vi "FileIO-Circular Wav Read.vi"(0 "Fileref in":T1, 5 "stimfileend":bool, 7 "Nread":i32, 9 "Loop?":bool, 11 "error in (no error)":errorcluster) -> (4 "Fileref out":T1, 6 "end of file?":bool, 8 "Y":dbl[](array[numeric]), 10 "looped":bool, 15 "error out":errorcluster)   [LabVIEW 2020]
uses:
  <vilib>/sound2/lvsound2.llb/Sound File Refnum.ctl
  <vilib>/sound2/lvsound2.llb/Sound File Position.ctl
  <vilib>/sound2/lvsound2.llb/Sound File Read (DBL).vi
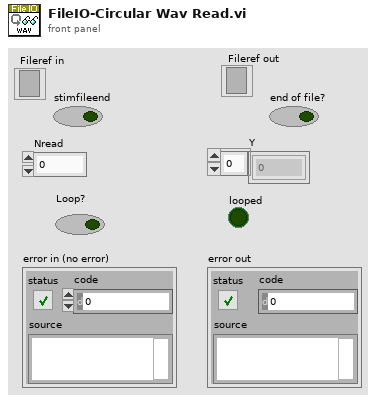
[diagram p1: front panel]
types:
  T1 = typedef "Sound File Refnum.ctl" = refnum<file>
  T2 = typedef "Sound File Position.ctl" = u16
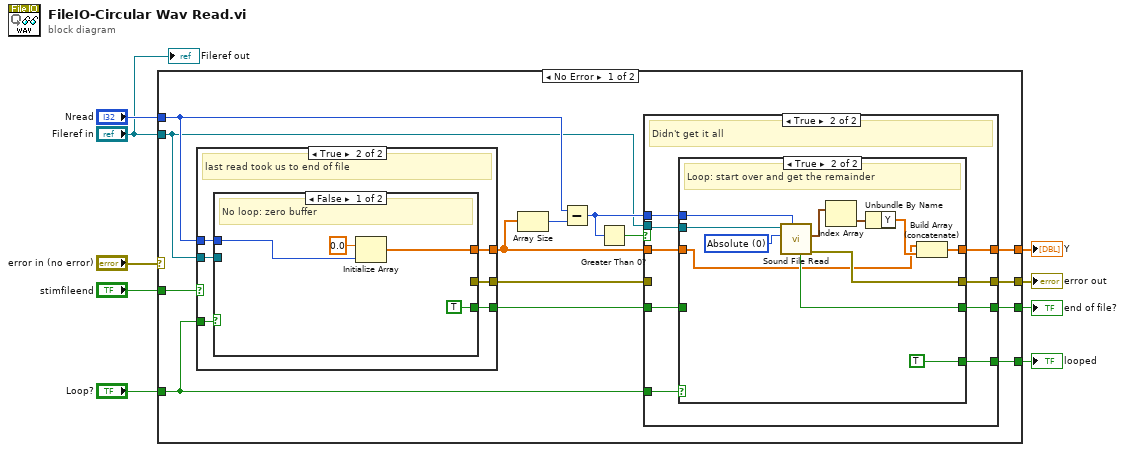
[diagram p0: block diagram]
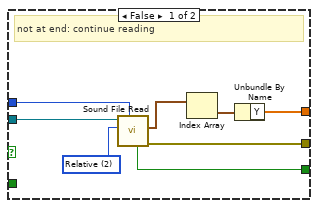
[diagram p2: hidden frame]
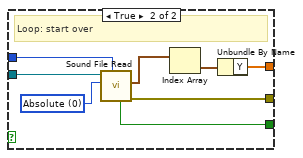
[diagram p3: hidden frame]
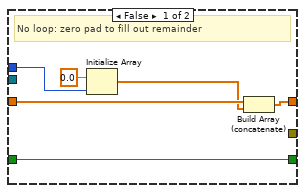
[diagram p5: hidden frame]
diagram:
  n1 = case shown="No Error" "error in (no error)" {
    selector: "error in (no error)" -> [_ w79]
    tunnel: "stimfileend" -> [w23 _]
    tunnel: "Nread" -> [w21 _]
    tunnel: "Fileref in" -> [w14 _]
    tunnel: "Loop?" -> [w13 _]
    tunnel: [w18 _] -> w4
    tunnel: [w16 w79] -> w3
    tunnel: [w11 _] -> w2
    tunnel: [w10 _] -> w1
    frame No Error {
      n2 = case shown="True" w23 {
        tunnel: [w26 w37] -> w17
        tunnel: w21 -> [w27 w36]
        tunnel: w14 -> [w28 w35]
        tunnel: w13 -> [_ w34]
        tunnel: [w25 w33] -> w19
        tunnel: [w24 w32] -> w12
        frame False {
          w31 = T2 2 items=["Absolute"=0, "Relative"=2] ("position mode")
          # "not at end: continue reading"
          n3 = call-poly <vilib>:"Sound File Read.vi"("number of samples/ch (-1: all)"=w27, "position mode"=w31, "sound file refnum"=w28) -> ("error out"=w26:errorcluster, "data"=w29:waveform(dbl)[], "end of file?"=w24:bool)  [unwired: 4 in, 2 out]
          n4 = Index Array(array=w29) -> (element=w30:waveform(dbl))  [unwired: 1 in]
          n5 = Unbundle By Name(w30) -> ("Y"=w25:dbl[])
        }
        frame True {
          # "last read took us to end of file"
          n6 = case shown="False" w34 {
            tunnel: [TRUE ("end of file?") w49] -> w32
            tunnel: [_ w48] -> w37
            tunnel: w36 -> [w41 w47]
            tunnel: w35 -> [_ w46]
            tunnel: [w39 w42] -> w33
            frame False {
              # "No loop: zero buffer"
              n7 = Initialize Array(0.0 ("element"), w41) -> (w39:dbl[])
            }
            frame True {
              w45 = T2 0 items=["Absolute"=0, "Relative"=2] ("position mode")
              # "Loop: start over"
              n8 = call-poly <vilib>:"Sound File Read.vi"("number of samples/ch (-1: all)"=w47, "position mode"=w45, "sound file refnum"=w46) -> ("error out"=w48:errorcluster, "data"=w43:waveform(dbl)[], "end of file?"=w49:bool)  [unwired: 4 in, 2 out]
              n9 = Index Array(array=w43) -> (element=w44:waveform(dbl))  [unwired: 1 in]
              n10 = Unbundle By Name(w44) -> ("Y"=w42:dbl[])
            }
          }
        }
      }
      n11 = Array Size(array=w19) -> (size(s)=w22:i32)
      n12 = Subtract(x=w21, y=w22) -> (x-y=w15:i32)
      n13 = Greater Than 0?(x=w15) -> (x > 0?=w20:bool)
      n14 = case shown="True" w20 {
        tunnel: w19 -> [w52 w59]
        tunnel: [w52 w58] -> w18
        tunnel: w17 -> [w51 _]
        tunnel: [w51 w54] -> w16
        tunnel: w15 -> [_ w60]
        tunnel: w14 -> [_ w55]
        tunnel: w13 -> [_ w61]
        tunnel: w12 -> [w50 w57]
        tunnel: [w50 w56] -> w11
        tunnel: [_ w53] -> w10
        frame False {
          # "Got it all. Do nothing."
        }
        frame True {
          # "Didn't get it all"
          n15 = case shown="True" w61 {
            tunnel: w60 -> [w67 w74]
            tunnel: w59 -> [w65 w70]
            tunnel: [w63 w69] -> w58
            tunnel: w57 -> [w62 _]
            tunnel: [w62 w72] -> w56
            tunnel: w55 -> [_ w75]
            tunnel: [_ w73] -> w54
            tunnel: [_ TRUE] -> w53
            frame False {
              # "No loop: zero pad to fill out remainder"
              n16 = Initialize Array(0.0 ("element"), w67) -> (w64:dbl[])
              n17 = Build Array (concatenate)(w65, w64) -> (w63:dbl[])
            }
            frame True {
              w78 = T2 0 items=["Absolute"=0, "Relative"=2] ("position mode")
              # "Loop: start over and get the remainder"
              n18 = call-poly <vilib>:"Sound File Read.vi"("number of samples/ch (-1: all)"=w74, "position mode"=w78, "sound file refnum"=w75) -> ("error out"=w73:errorcluster, "data"=w76:waveform(dbl)[], "end of file?"=w72:bool)  [unwired: 4 in, 2 out]
              n19 = Index Array(array=w76) -> (element=w77:waveform(dbl))  [unwired: 1 in]
              n20 = Unbundle By Name(w77) -> ("Y"=w71:dbl[])
              n21 = Build Array (concatenate)(w70, w71) -> (w69:dbl[])
            }
          }
        }
      }
    }
    frame Error {
    }
  }
  "end of file?" <- w2
  "Y" <- w4
  "error out" <- w3
  "looped" <- w1
  "Fileref out" <- "Fileref in"
